vi "LH_TailPopListNode.vi"(0 "InputList":refnum<class "ListHead.lvclass">) -> (1 "OutputList":refnum<class "ListHead.lvclass">, 2 "Content":u32, 3 "IsEmpty?":bool)   [LabVIEW 2014, in "ListHead.lvclass"]
uses:
  ListHead.lvclass
  ListHead.lvclass/ListHead.ctl
  ListNode.lvclass
  ListNodeVirtual.lvclass
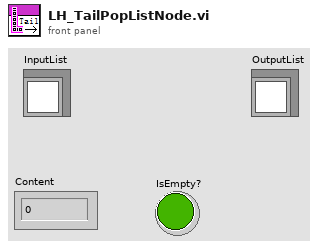
[diagram p1: front panel]
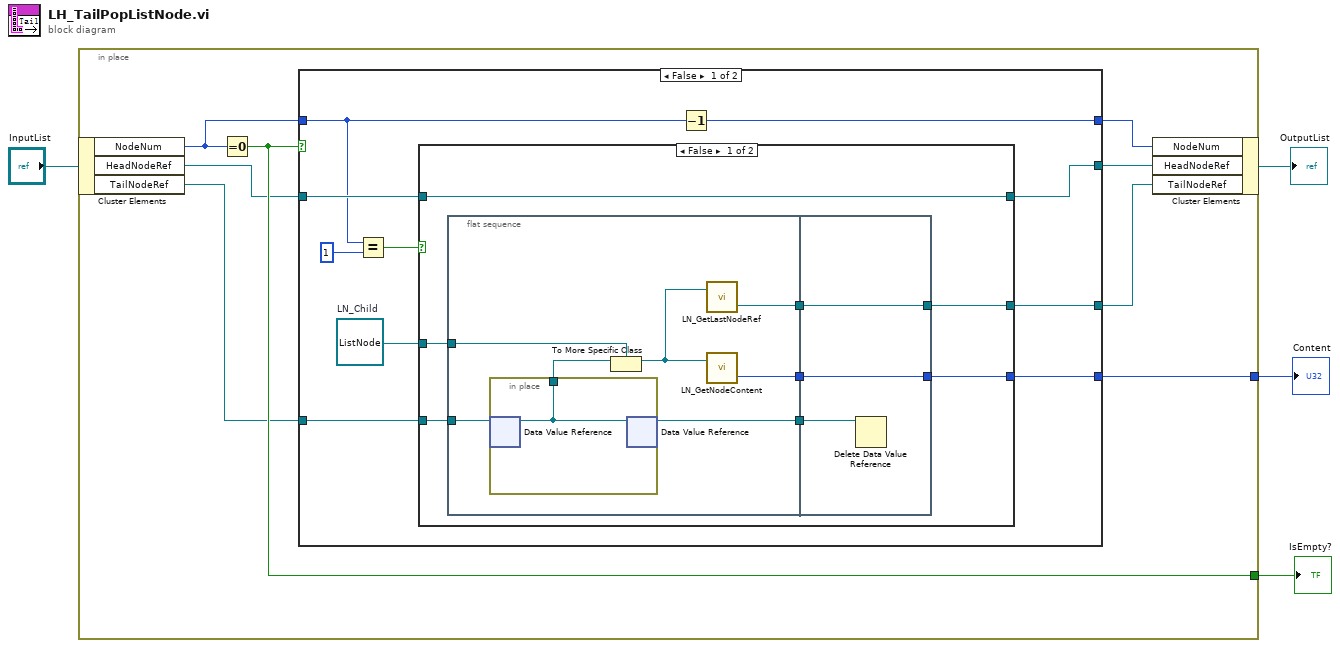
[diagram p0: block diagram]
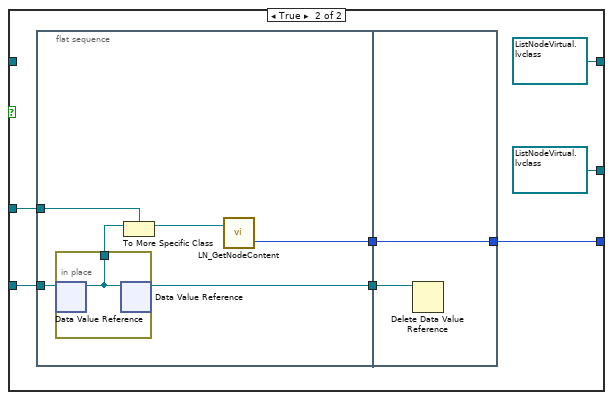
[diagram p2: hidden frame]
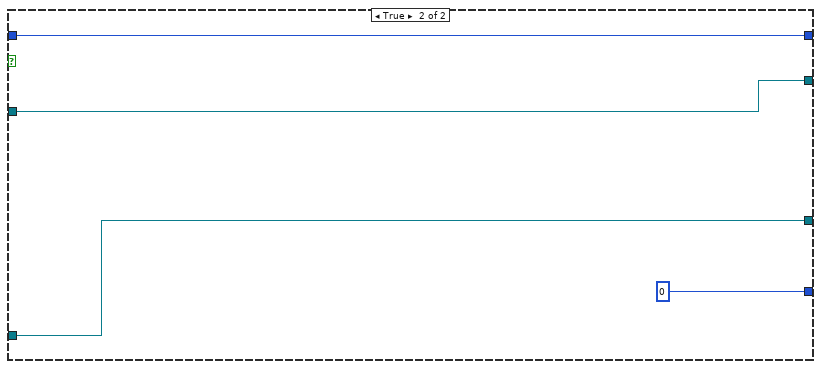
[diagram p3: hidden frame]
diagram:
  n1 = in-place {
    in-place-border: [w11] -> w2
    in-place-border: [w7] -> w1
    n2 = in-place-cluster #1("InputList") -> ("NodeNum"=w12:u32, "HeadNodeRef"=w9:refnum<data-value>, "TailNodeRef"=w8:refnum<data-value>)
    n3 = Equal To 0?(x=w12) -> (x = 0?=w11:bool)
    n4 = case shown="False" w11 {
      tunnel: w12 -> [w18 w61]
      tunnel: [w22 w61] -> w10
      tunnel: w9 -> [w21 w59]
      tunnel: w8 -> [w20 w58]
      tunnel: [w16 u32 0] -> w7
      tunnel: [w15 w58] -> w6
      tunnel: [w14 w59] -> w5
      frame False {
        w13 = refnum<class "ListNode.lvclass"> refnum  # LN_Child
        n5 = Equal?(x=w18, y=u32 1) -> (x = y?=w19:bool)
        n6 = case shown="False" w19 {
          tunnel: w21 -> [w24 _]
          tunnel: w20 -> [w30 w48]
          tunnel: [w29 w45] -> w16
          tunnel: [w25 refnum<data-value> refnum ("OutputLastNodeRef")] -> w15
          tunnel: [w24 refnum<data-value> refnum ("HeadNodeRef")] -> w14
          tunnel: w13 -> [w23 w47]
          frame False {
            n7 = flat-sequence {
              tunnel: w30 -> [w32]
              tunnel: [w36] -> w28
              tunnel: [w35] -> w27
              tunnel: [w34] -> w26
              tunnel: w23 -> [w33]
              tunnel: [w41] -> w29
              tunnel: w28 -> [w41]
              tunnel: w27 -> [w40]
              tunnel: [w39] -> w25
              tunnel: w26 -> [w39]
              frame #0 {
                n8 = in-place {
                  in-place-border: [w38] -> w37
                  n9 = in-place-dvr #2(w32) -> (w38:refnum<class "ListNodeVirtual.lvclass">)  [unwired: 1 out]
                  n10 = in-place-dvr #2(w38) -> (w35:refnum<data-value>)  [unwired: 1 out]
                }
                n11 = To More Specific Class(target class=w33, reference=w37) -> (specific class reference=w31:refnum<class "ListNode.lvclass">)  [unwired: 1 in, 1 out]
                n12 = call "LN_GetLastNodeRef.vi"("InputListNode"=w31) -> ("OutputLastNodeRef"=w34:refnum<data-value>)  [unwired: 1 in, 1 out]
                n13 = call "LN_GetNodeContent.vi"("InputNode"=w31) -> ("Content"=w36:i32)  [unwired: 1 in, 1 out]
              }
              frame #1 {
                n14 = Delete Data Value Reference(data value reference=w40) -> ()  [unwired: 1 in, 2 out]
              }
            }
          }
          frame True {
            n15 = flat-sequence {
              tunnel: w48 -> [w54]
              tunnel: w47 -> [w53]
              tunnel: [w50] -> w46
              tunnel: [w49] -> w44
              tunnel: w46 -> [w57]
              tunnel: [w57] -> w45
              tunnel: w44 -> [w56]
              frame #0 {
                n16 = in-place {
                  in-place-border: [w55] -> w52
                  n17 = in-place-dvr #3(w54) -> (w55:refnum<class "ListNodeVirtual.lvclass">)  [unwired: 1 out]
                  n18 = in-place-dvr #3(w55) -> (w49:refnum<data-value>)  [unwired: 1 out]
                }
                n19 = To More Specific Class(target class=w53, reference=w52) -> (specific class reference=w51:refnum<class "ListNode.lvclass">)  [unwired: 1 in, 1 out]
                n20 = call "LN_GetNodeContent.vi"("InputNode"=w51) -> ("Content"=w50:i32)  [unwired: 1 in, 1 out]
              }
              frame #1 {
                n21 = Delete Data Value Reference(data value reference=w56) -> ()  [unwired: 1 in, 2 out]
              }
            }
          }
        }
        n22 = Decrement(x=w18) -> (x-1=w22:u32)
      }
      frame True {
      }
    }
    n23 = in-place-cluster #1("NodeNum"=w10, "HeadNodeRef"=w5, "TailNodeRef"=w6) -> (→"OutputList":refnum<class "ListHead.lvclass">)
  }
  "IsEmpty?" <- w2
  "Content" <- w1
